vi "buildscript.vi"() -> ()   [LabVIEW 2021]
uses:
  Application_class/Application.lvclass
  CetoniPump_class/CetoniPump.lvclass
  <vilib>/Utility/config.llb/NI_LVConfig.lvlib
panel:
  out "key-value 2":variant
  out "key-value":variant
  in  "Go to Level 3":T1
  in  "Exit":bool
  in  "Inject Error<Replace Me>":bool
  in  "Go to Level 2":T1
  in  "Go to Level":bool
  in  "Syringe":T2(ring)=enum."BD 5ml"
  out "Syringe Helper":T3={"Maximum Piston Stroke (mm)"=48.147993421803335, "Inner Diameter (mm)"=12.06}
  in  "Stop ALL Pumps":bool
  in  "ConfigureSyringe":bool
  in  "SyringeSettings":T4={"index"=0, "SyringeSettings"={"Maximum Piston Stroke (mm)"=100.0, "Inner Diameter (mm)"=12.0}}
  in  "ReadStatus":bool
  in  "ReferenceMove":bool
  in  "Do Something <Replace Me>":bool
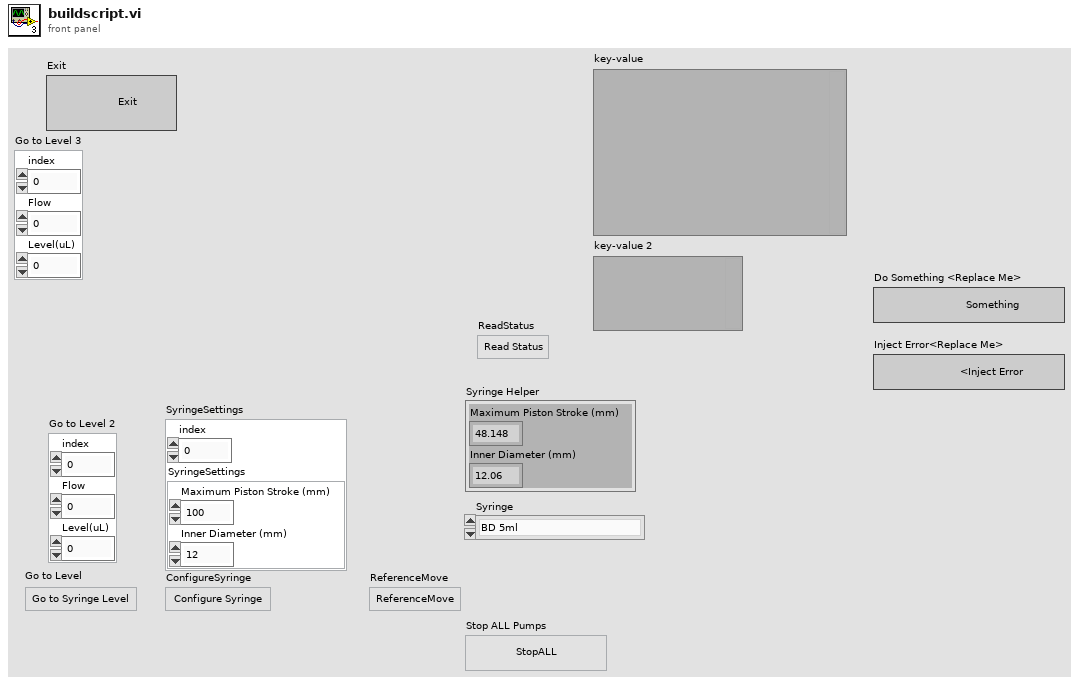
[diagram p1: front panel]
types:
  T1 = cluster{"index":i32, "Flow":dbl, "Level(uL)":dbl}
  T2 = enum16{"BD 1ml", "BD 3ml", "BD 5ml", "BD 10ml", "BD 20ml", "BD 30ml", "BD 50ml", "HSW 1ml"}
  T3 = cluster{"Maximum Piston Stroke (mm)":dbl, "Inner Diameter (mm)":dbl}
  T4 = cluster{"index":i32, "SyringeSettings":cluster{"Maximum Piston Stroke (mm)":dbl, "Inner Diameter (mm)":dbl}}
  T5 = cluster{"Message":string, "Message Data":variant}[]
  T6 = typedef "NI_LVConfig.lvlib/Config Data RefNum.ctl" = refnum<k1>
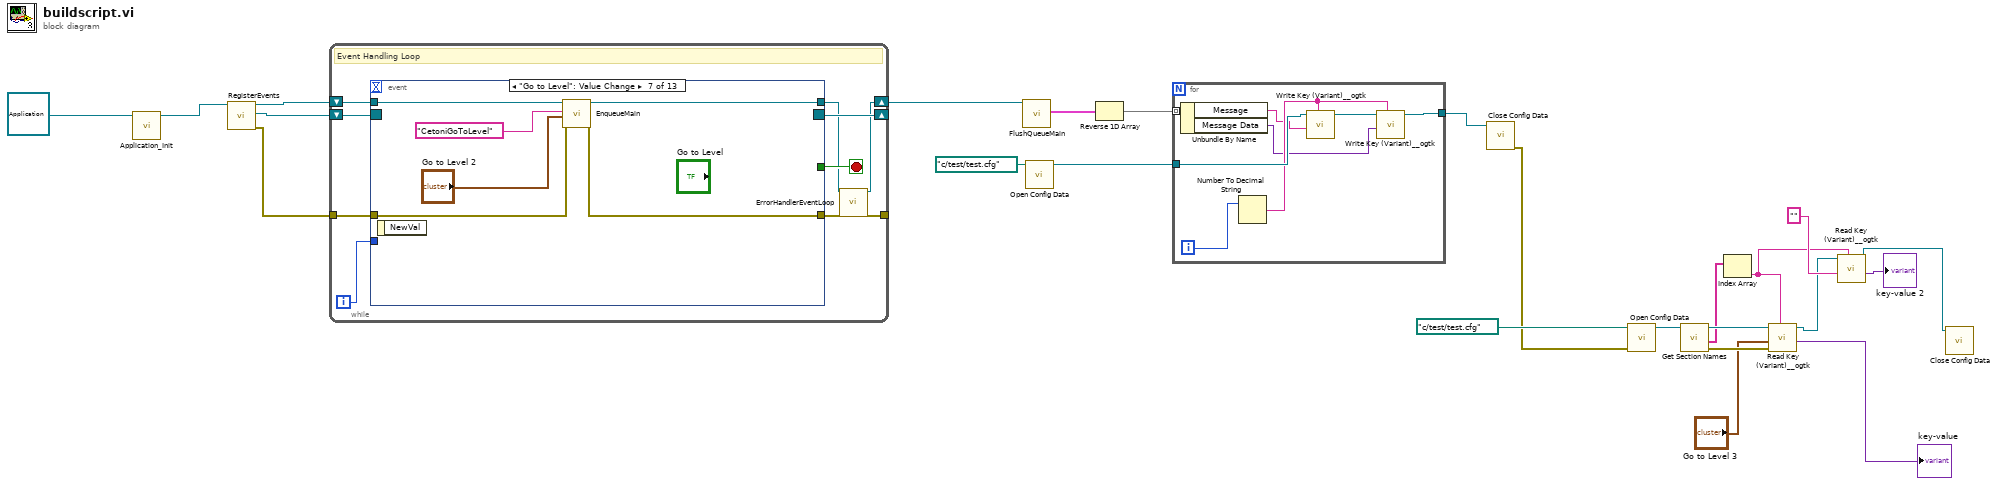
[diagram p0: block diagram]
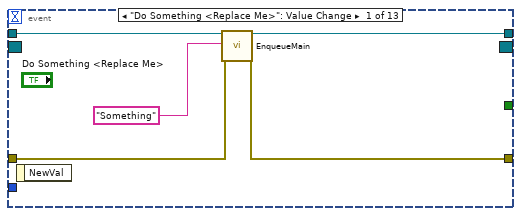
[diagram p2: hidden frame]
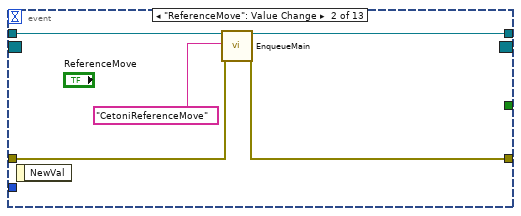
[diagram p3: hidden frame]
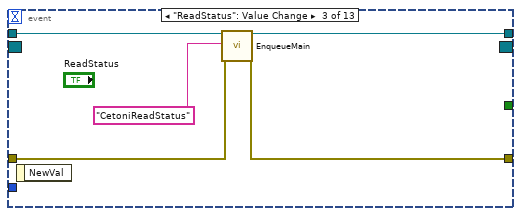
[diagram p4: hidden frame]
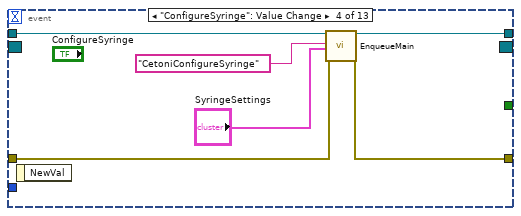
[diagram p5: hidden frame]
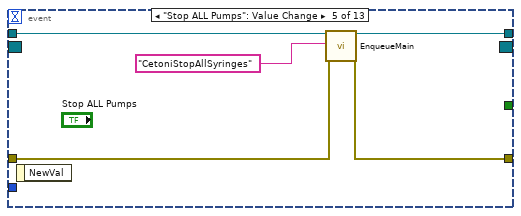
[diagram p6: hidden frame]
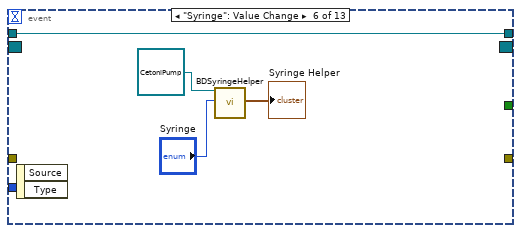
[diagram p7: hidden frame]
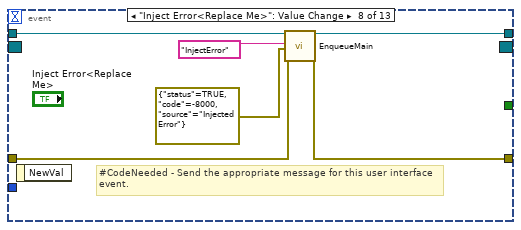
[diagram p8: hidden frame]
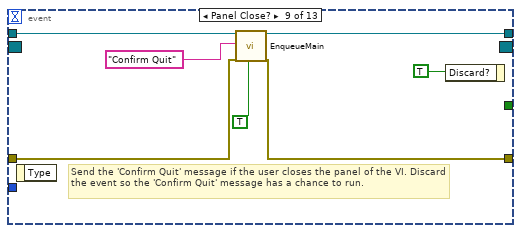
[diagram p9: hidden frame]
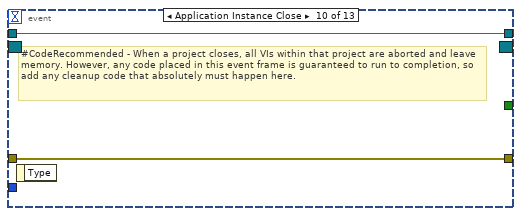
[diagram p10: hidden frame]
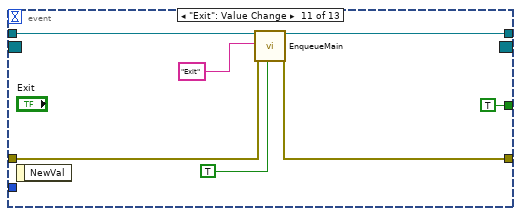
[diagram p11: hidden frame]
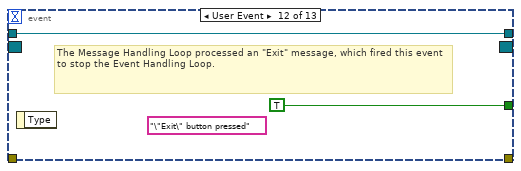
[diagram p12: hidden frame]
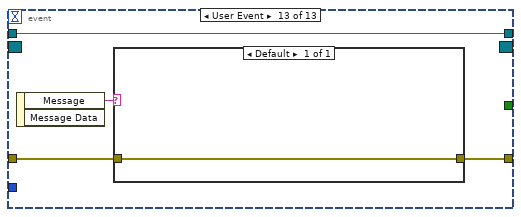
[diagram p13: hidden frame]
diagram:
  n1 = call "Application_Init.vi"("object in"=refnum<class "Application.lvclass"> refnum ("Application")) -> ("object out"=w20:refnum<class "Application.lvclass">)  [unwired: 17 in, 1 out]
  n2 = call-dynamic "RegisterEvents.vi"("object in"=w20) -> ("object out"=w24:refnum<class "Application.lvclass">, "Event Registration Refnum"=w23:refnum<event-registration>, "error out"=w22:errorcluster)  [unwired: 16 in]
  n3 = while {
    shift-right: [w33] -> _
    shift-left: w23 -> [w34]
    tunnel: [w28] -> _
    shift-right: [w26] -> w18
    shift-left: w24 -> [w31]
    tunnel: w22 -> [w30]
    i -> [w25]
    stop <- w32 stop-if-true
    # "Event Handling Loop"
    n4 = event shown="[6] \"Go to Level\": Value Change" {
      selector: w34 -> [_ _ _ _ _ _ _ _ _ _ _ _ _]
      dyn-events: [_ _ _ _ _ _ _ _ _ _ _ _ _] -> w33
      timeout: _ -> [_ _ _ _ _ _ _ _ _ _ _ _ _]
      tunnel: [_ _ _ _ _ _ _ _ _ _ TRUE ("Discard?") TRUE ("Discard?") _] -> w32
      tunnel: [w36 w41 w46 w53 w57 _ w67 w73 w79 w84 w87 _ w95] -> w29
      tunnel: w31 -> [w39 w44 w49 w55 w60 w64 w70 w76 w78 w85 w92 w93 w98]
      tunnel: [w38 w43 w48 w54 w59 w64 w69 w75 w77 w85 w91 w93 w98] -> w27
      tunnel: w30 -> [w35 w40 w45 w52 w56 _ w66 w72 w80 w84 w88 _ w96]
      tunnel: w25 -> [_ _ _ _ _ _ _ _ _ _ _ _ _]
      event "Do Something <Replace Me>": Value Change {
        n5 = event-data() -> ()  [unwired: 1 in, 1 out]
        n6 = call-dynamic "EnqueueMain.vi"("object in"=w39, "Message"="Something", "error in (no error)"=w35) -> ("object out"=w38:refnum<class "Application.lvclass">, "error out"=w36:errorcluster)  [unwired: 15 in]
      }
      event "ReferenceMove": Value Change {
        n7 = event-data() -> ()  [unwired: 1 in, 1 out]
        n8 = call-dynamic "EnqueueMain.vi"("object in"=w44, "Message"="CetoniReferenceMove", "error in (no error)"=w40) -> ("object out"=w43:refnum<class "Application.lvclass">, "error out"=w41:errorcluster)  [unwired: 15 in]
      }
      event "ReadStatus": Value Change {
        n9 = event-data() -> ()  [unwired: 1 in, 1 out]
        n10 = call-dynamic "EnqueueMain.vi"("object in"=w49, "Message"="CetoniReadStatus", "error in (no error)"=w45) -> ("object out"=w48:refnum<class "Application.lvclass">, "error out"=w46:errorcluster)  [unwired: 15 in]
      }
      event "ConfigureSyringe": Value Change {
        n11 = event-data() -> ()  [unwired: 1 in, 1 out]
        n12 = call-dynamic "EnqueueMain.vi"("object in"=w55, "Message"="CetoniConfigureSyringe", "Message Data"="SyringeSettings", "error in (no error)"=w52) -> ("object out"=w54:refnum<class "Application.lvclass">, "error out"=w53:errorcluster)  [unwired: 14 in]
      }
      event "Stop ALL Pumps": Value Change {
        n13 = event-data() -> ()  [unwired: 1 in, 1 out]
        n14 = call-dynamic "EnqueueMain.vi"("object in"=w60, "Message"="CetoniStopAllSyringes", "error in (no error)"=w56) -> ("object out"=w59:refnum<class "Application.lvclass">, "error out"=w57:errorcluster)  [unwired: 15 in]
      }
      event "Syringe": Value Change {
        n15 = event-data() -> ()  [unwired: 1 in, 2 out]
        n16 = call-dynamic "BDSyringeHelper.vi"("object in"=refnum<class "CetoniPump.lvclass"> refnum, "Syringe"="Syringe") -> ("output cluster"=→"Syringe Helper":T3)  [unwired: 15 in, 2 out]
      }
      event "Go to Level": Value Change {
        n17 = event-data() -> ()  [unwired: 1 in, 1 out]
        n18 = call-dynamic "EnqueueMain.vi"("object in"=w70, "Message"="CetoniGoToLevel", "Message Data"="Go to Level 2", "error in (no error)"=w66) -> ("object out"=w69:refnum<class "Application.lvclass">, "error out"=w67:errorcluster)  [unwired: 14 in]
      }
      event "Inject Error<Replace Me>": Value Change {
        # "#CodeNeeded - Send the appropriate message for this user interface event."
        n19 = event-data() -> ()  [unwired: 1 in, 1 out]
        n20 = call-dynamic "EnqueueMain.vi"("object in"=w76, "Message"="InjectError", "Message Data"=errorcluster {"status"=TRUE, "code"=-8000, "source"="Injected Error"} ("error in (no error)"), "error in (no error)"=w72) -> ("object out"=w75:refnum<class "Application.lvclass">, "error out"=w73:errorcluster)  [unwired: 14 in]
      }
      event Panel Close? {
        # "Send the 'Confirm Quit' message if the user closes the panel of the VI. Discard the event so the 'Confirm Quit' message has a chance to run."
        n21 = event-data() -> ()  [unwired: 1 in, 1 out]
        n22 = call-dynamic "EnqueueMain.vi"("object in"=w78, "Message"="Confirm Quit", "error in (no error)"=w80, "Priority Message? (F)"=TRUE) -> ("object out"=w77:refnum<class "Application.lvclass">, "error out"=w79:errorcluster)  [unwired: 14 in]
        n23 = event-data("Discard?"=TRUE) -> ()  [unwired: 1 in, 1 out]
      }
      event Application Instance Close {
        # "#CodeRecommended - When a project closes, all VIs within that project are aborted and leave memory. However, any code placed in this event frame is guaranteed to run to completion, so add any cleanup code that absolutely must happen here."
        n24 = event-data() -> ()  [unwired: 1 in, 1 out]
      }
      event "Exit": Value Change {
        n25 = event-data() -> ()  [unwired: 1 in, 1 out]
        n26 = call-dynamic "EnqueueMain.vi"("object in"=w92, "Message"="Exit", "error in (no error)"=w88, "Priority Message? (F)"=TRUE) -> ("object out"=w91:refnum<class "Application.lvclass">, "error out"=w87:errorcluster)  [unwired: 14 in]
      }
      event User Event {
        (unwired) "\"Exit\" button pressed" ("VI Stopped")
        # "The Message Handling Loop processed an \"Exit\" message, which fired this event to stop the Event Handling Loop."
        n27 = event-data() -> ()  [unwired: 1 in, 1 out]
      }
      event User Event {
        n28 = event-data() -> ("Message"=w97:string)  [unwired: 1 in, 1 out]
        n29 = case shown="Default" w97 {
          tunnel: w96 -> [w99]
          tunnel: [w99] -> w95
          frame Default {
          }
        }
      }
    }
    n30 = call-dynamic "ErrorHandlerEventLoop.vi"("object in"=w27, "error in (no error)"=w29) -> ("object out"=w26:refnum<class "Application.lvclass">, "error out"=w28:errorcluster)  [unwired: 16 in]
  }
  n31 = call-dynamic "FlushQueueMain.vi"("object in"=w18) -> ("remaining elements"=w15:T5)  [unwired: 16 in, 2 out]
  n32 = call <vilib>:"Open Config Data.vi"("configuration file path"=path "c:/test/test.cfg") -> ("refnum"=w17:T6)  [unwired: 8 in, 2 out]
  n33 = Reverse 1D Array(array=w15) -> (reversed array=w14:T5)
  n34 = for {
    tunnel: w14 -> [w107] mode=indexing
    tunnel: w17 -> [w105]
    tunnel: [w103] -> w16
    i -> [w106]
    n35 = Unbundle By Name(w107) -> ("Message"=w100:string, "Message Data"=w101:variant)
    n36 = Number To Decimal String(number=w106) -> (decimal integer string=w102:string)  [unwired: 1 in]
    n37 = call <userlib>:"Write Key (Variant)__ogtk.vi"("section"=w102, "key-value"=w100, "refnum"=w105) -> ("refnum out"=w104:T6)  [unwired: 7 in, 1 out]
    n38 = call <userlib>:"Write Key (Variant)__ogtk.vi"("section"=w102, "key-value"=w101, "refnum"=w104) -> ("refnum out"=w103:T6)  [unwired: 7 in, 1 out]
  }
  n39 = call <vilib>:"Close Config Data.vi"("refnum"=w16) -> ("error out"=w12:errorcluster)  [unwired: 9 in, 1 out]
  n40 = call <vilib>:"Open Config Data.vi"("error in (no error)"=w12, "configuration file path"=path "c:/test/test.cfg") -> ("refnum"=w11:T6)  [unwired: 7 in, 2 out]
  n41 = call <vilib>:"Get Section Names.vi"("refnum"=w11) -> ("error out"=w8:errorcluster, "section names"=w9:string[], "refnum out"=w10:T6)  [unwired: 8 in]
  n42 = Index Array(array=w9) -> (element=w4:string)  [unwired: 1 in]
  n43 = call <userlib>:"Read Key (Variant)__ogtk.vi"("section"=w4, "error in (no error)"=w8, "type"="Go to Level 3", "refnum"=w10) -> ("key-value"=→"key-value":variant, "refnum out"=w2:T6)  [unwired: 4 in, 2 out]
  n44 = call <userlib>:"Read Key (Variant)__ogtk.vi"("section"=w4, "type"="" ("Message"), "refnum"=w2) -> ("key-value"=→"key-value 2":variant, "refnum out"=w1:T6)  [unwired: 5 in, 2 out]
  n45 = call <vilib>:"Close Config Data.vi"("refnum"=w1) -> ()  [unwired: 9 in, 2 out]
